vi "lv-saveAndCloseProject.vi"(8 "error in (no error)":errorcluster, 11 "Project refs":T1={"LabVIEW Project Path"=path "C:/Users/admin/Desktop/Source/Waveform-Processing-Custom-Device.lvproj", "Project refnum"=refnum, "Build spec refnum"=refnum}) -> (0 "error out":errorcluster={"status"=TRUE, "code"=7, "source"="Invoke Node in InstallerBuildSpec.OpenReference.vi\n<APPEND>\nMethod Name: <b>Project:Open</b>"})   [LabVIEW 2014, in "veristand-steps-build-system.lvlib"]
uses:
  veristand-steps-build-system.lvlib
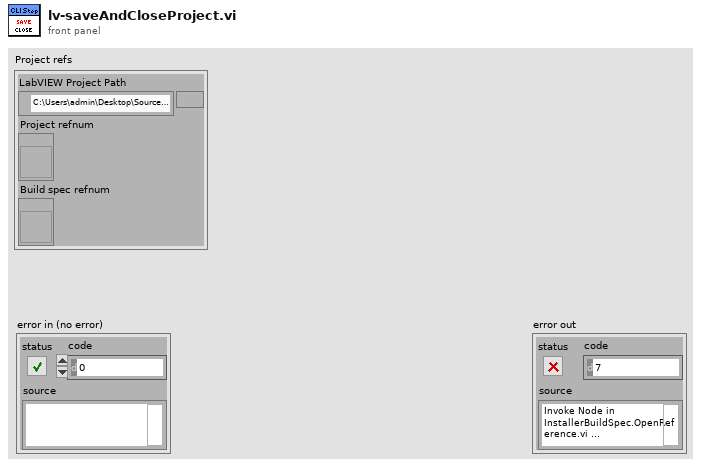
[diagram p1: front panel]
types:
  T1 = cluster{"LabVIEW Project Path":path, "Project refnum":refnum<vi>, "Build spec refnum":refnum<vi>}
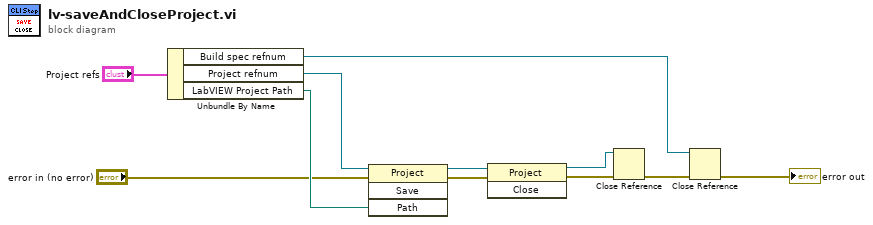
[diagram p0: block diagram]
diagram:
  n1 = Unbundle By Name("Project refs") -> ("Build spec refnum"=w3:refnum<vi>, "Project refnum"=w4:refnum<vi>, "LabVIEW Project Path"=w2:path)
  n2 = invoke class="Project" method="Save"(reference=w4, error in="error in (no error)", "Path"=w2) -> (reference out=w6:refnum<vi>, error out=w7:errorcluster)  [unwired: 1 in, 2 out]
  n3 = invoke class="Project" method="Close"(reference=w6, error in=w7) -> (reference out=w10:refnum<vi>, error out=w8:errorcluster)  [unwired: 1 in, 1 out]
  n4 = Close Reference(reference=w10, error in (no error)=w8) -> (error out=w9:errorcluster)
  n5 = Close Reference(reference=w3, error in (no error)=w9) -> (error out=→"error out":errorcluster)
